vi "Error Queue - Enqueue Element.vi"(8 "error in (no error)":errorcluster, 11 "Error Queue IN":refnum<queue>) -> (0 "error out":errorcluster)   [LabVIEW 2019]
panel:
  # "--- Inputs ---"
  # "--- Outputs ---"
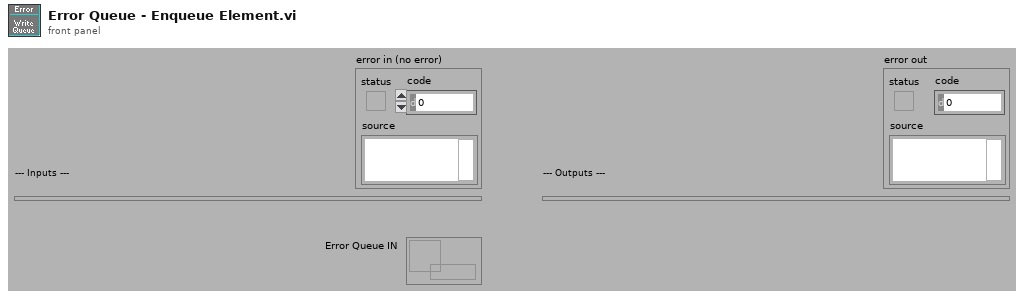
[diagram p1: front panel]
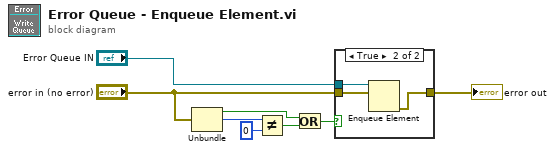
[diagram p0: block diagram]
diagram:
  n1 = Unbundle("error in (no error)") -> ("status"=w3:bool, "code"=w6:i32)  [unwired: 1 out]
  n2 = Not Equal?(x=w6, y=0) -> (x != y?=w4:bool)
  n3 = Or(x=w3, y=w4) -> (x .or. y?=w2:bool)
  n4 = case shown="True" w2 {
    tunnel: "Error Queue IN" -> [_ w12]
    tunnel: "error in (no error)" -> [w9 w11]
    tunnel: [w9 w10] -> w8
    frame False {
    }
    frame True {
      n5 = Enqueue Element(queue=w12, element=w11) -> (error out=w10:errorcluster)  [unwired: 2 in, 2 out]
    }
  }
  "error out" <- w8
